vi "sendUpdateCommand.vi"(8 "error in (no error)":errorcluster, 10 "model":refnum<class "Model.lvclass">, 11 "FaultState in":refnum<class "FaultState.lvclass">) -> (0 "error out":errorcluster, 2 "model 2":refnum<class "Model.lvclass">, 3 "FaultState out":refnum<class "FaultState.lvclass">)   [LabVIEW 2013, in "FaultState.lvclass"]
uses:
  FaultState.lvclass
  Model/Model/Model.lvclass
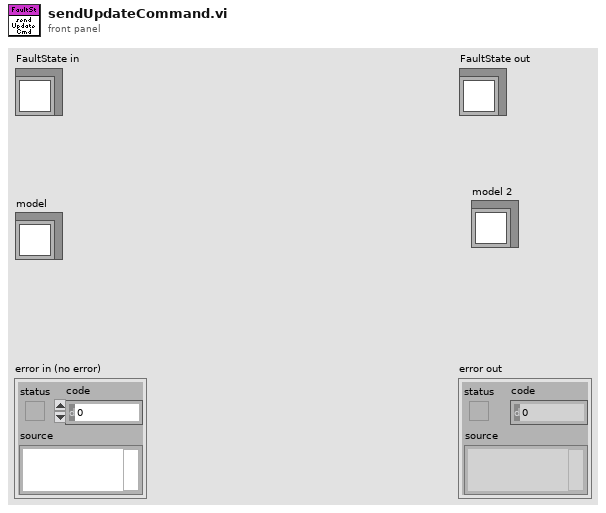
[diagram p1: front panel]
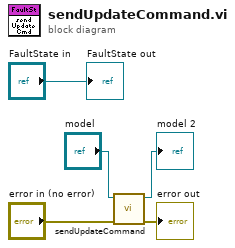
[diagram p0: block diagram]
diagram:
  n1 = call "sendUpdateCommand.vi"("error in (no error)"="error in (no error)", "Model in"="model") -> ("error out"=→"error out":errorcluster, "Model out"=→"model 2":refnum<class "Model.lvclass">)  [unwired: 8 in]
  "FaultState out" <- "FaultState in"
